vi "New Prop B.vi"(11 "GIC Input":T1={"     Use ?\nOff       On"=[FALSE, TRUE, FALSE, TRUE], "Mode:"=FALSE, "WP Data"="", "Hokuyo Port"="COM7", "Prop  Port"="COM6", "Compass Port"="", "GPS Port"="", "Num of WPs"=0, "WP Lats and Longs"={"WP Lats"=[], "WP Longs"=[]}, "Obst Lats and Longs"={"Obst Lats"=[], "Obst Longs"=[]}, "Parameters"=[], "GPS Data"=[], "Compass"=0.0, "LMS Vector"=[], "Vision Vector"=[], "Direction Cmd"=0.0, "Speed Cmd"=0.0, "WP Vector"=[], "WP Number"=0, "Extra"=0, "SW Map"=[], "Path Cluster"={"Path x node"=[], "Path y node"=[]}} {"Obst Lats and Longs"."Obst Longs" format="%#_8g"; "Obst Lats and Longs"."Obst Lats" format="%#_8g"}) -> ()   [LabVIEW 2014]
uses:
  <vilib>/Instr/_visa.llb/VISA Configure Serial Port (Instr).vi
panel:
  out "Prop VISA Resource Name":refnum<visa-resource-name>
  # "New Prop B"
  # "Input:"
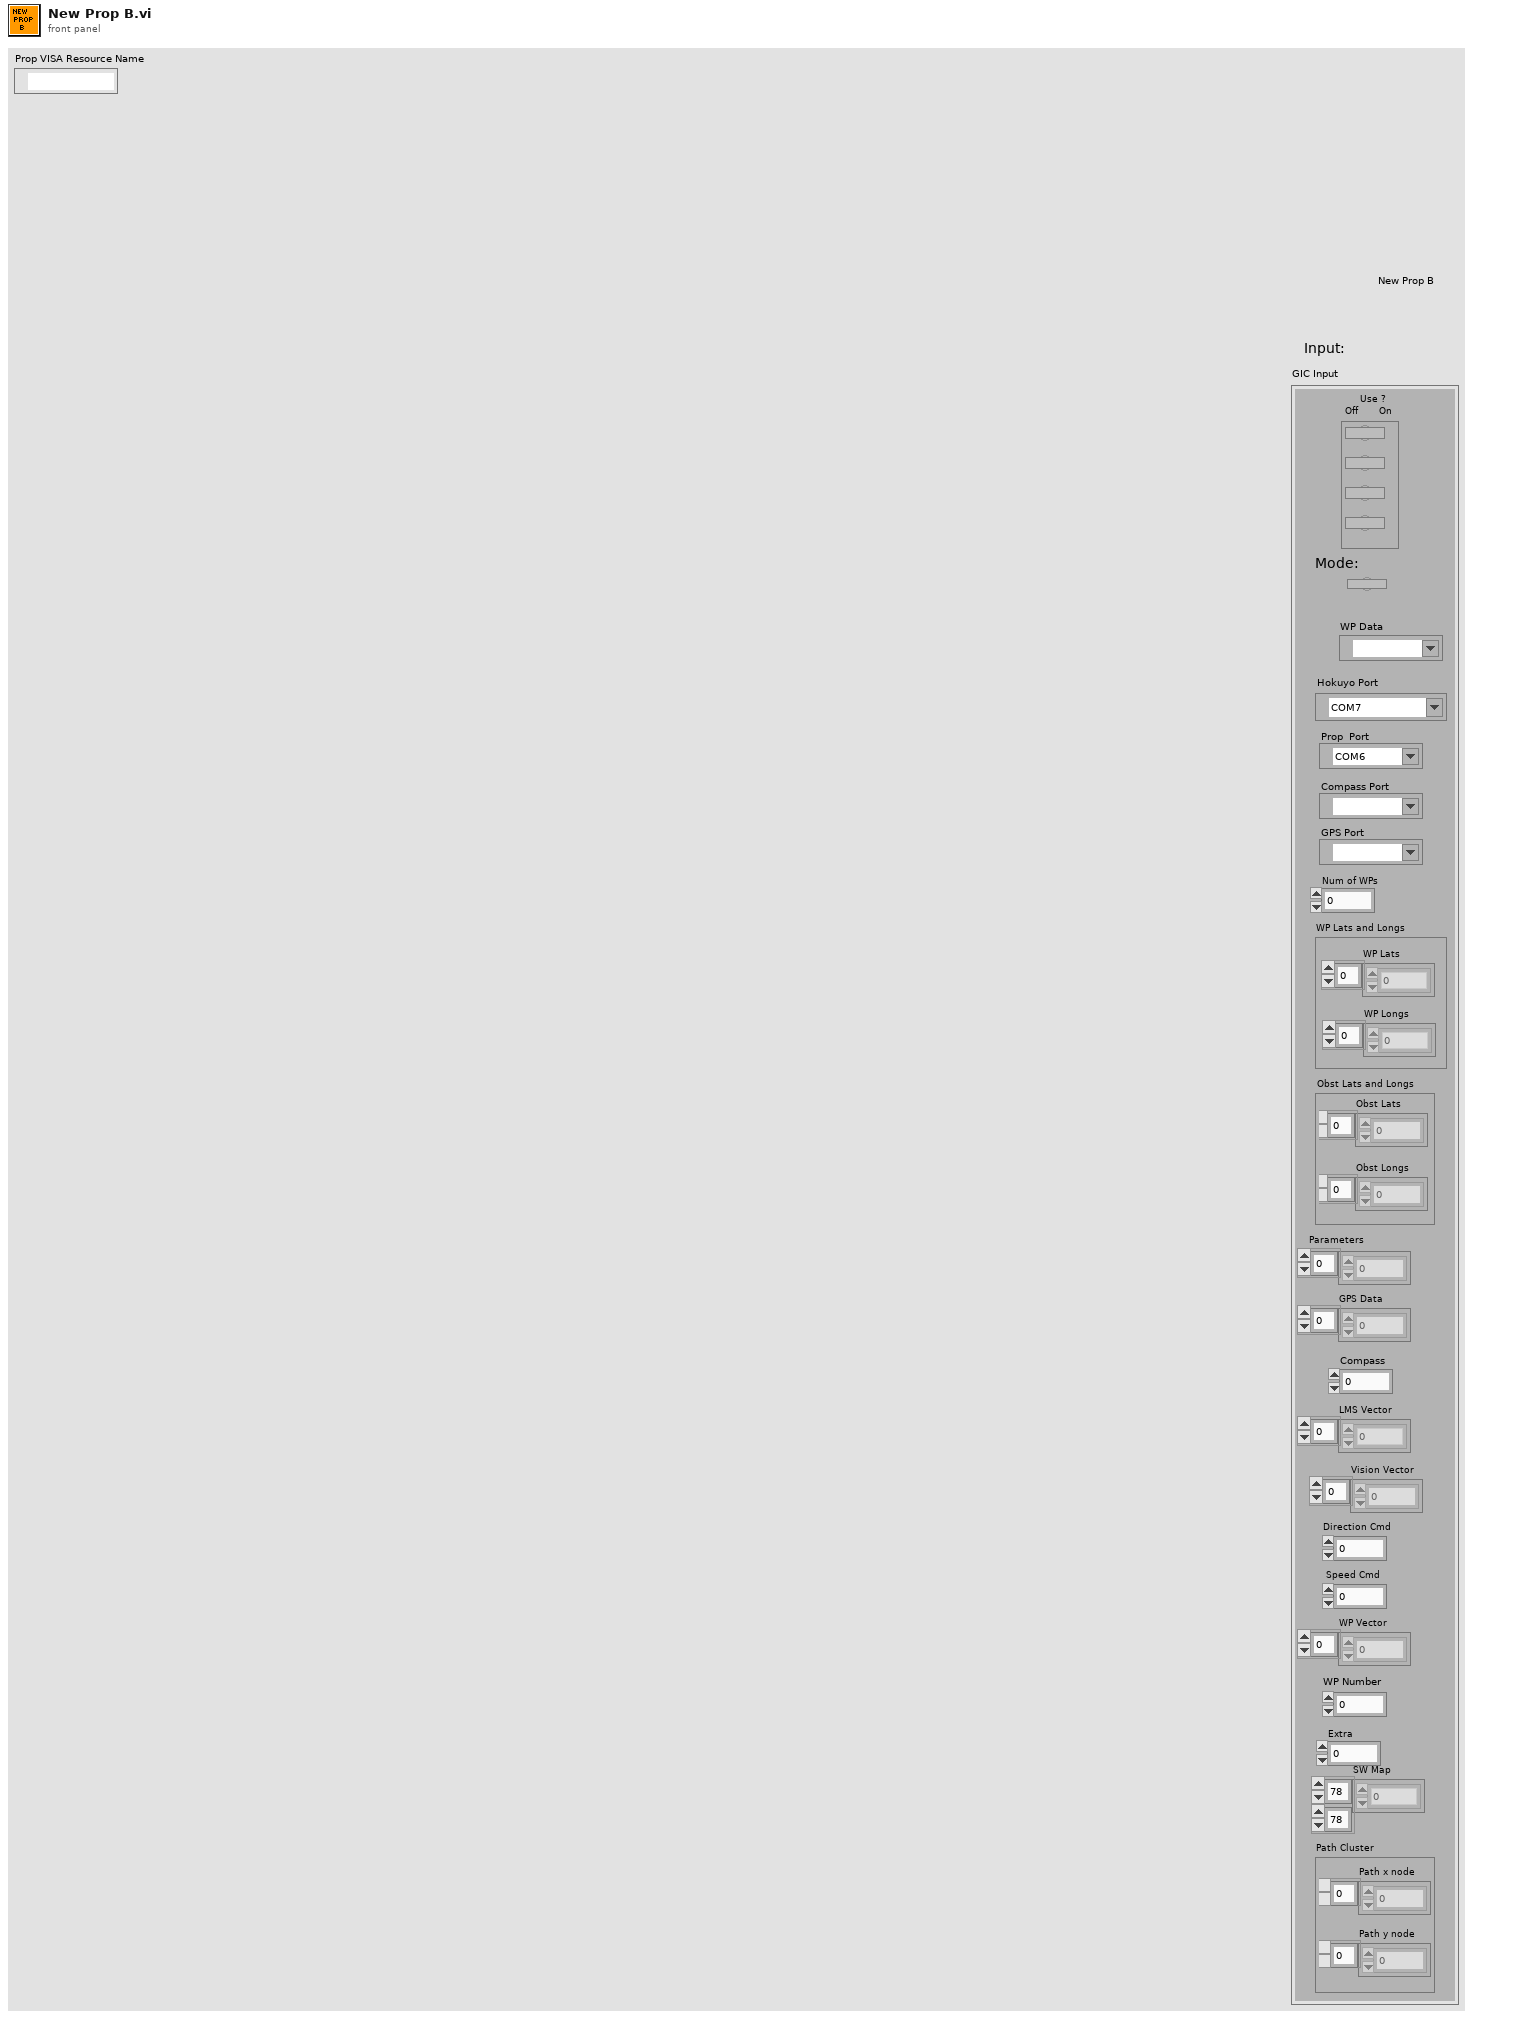
[diagram p1: front panel]
types:
  T1 = cluster{"     Use ?\nOff       On":bool[], "Mode:":bool, "WP Data":refnum<visa-resource-name>, "Hokuyo Port":refnum<visa-resource-name>, "Prop  Port":refnum<visa-resource-name>, "Compass Port":refnum<visa-resource-name>, "GPS Port":refnum<visa-resource-name>, "Num of WPs":i16, "WP Lats and Longs":cluster{"WP Lats":dbl[], "WP Longs":dbl[]}, "Obst Lats and Longs":cluster{"Obst Lats":dbl[], "Obst Longs":dbl[]}, "Parameters":dbl[], "GPS Data":dbl[], "Compass":dbl, "LMS Vector":dbl[], "Vision Vector":dbl[], "Direction Cmd":dbl, "Speed Cmd":dbl, "WP Vector":dbl[], "WP Number":i32, "Extra":i16, "SW Map":i32[][], "Path Cluster":cluster{"Path x node":dbl[], "Path y node":dbl[]}}
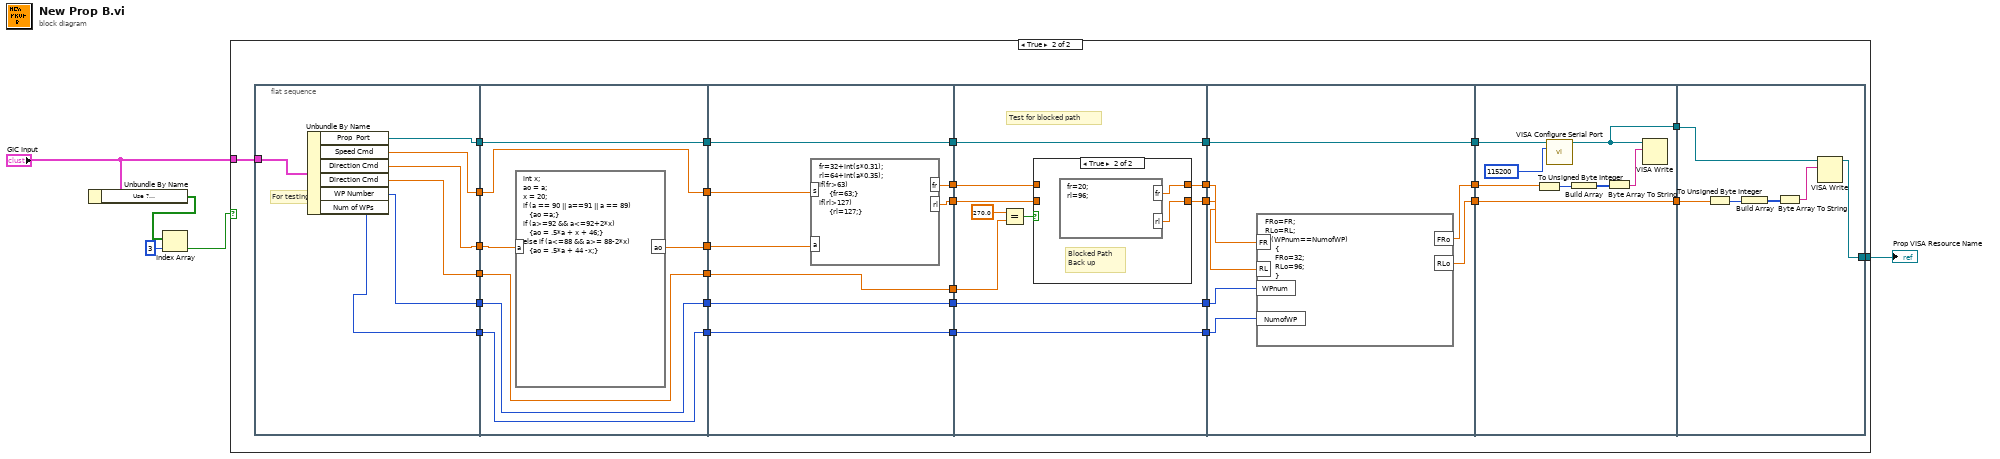
[diagram p0: block diagram]
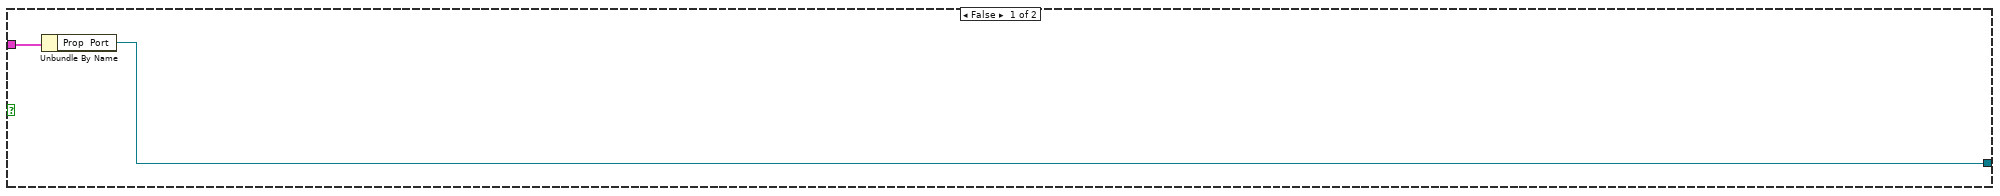
[diagram p2: hidden frame]
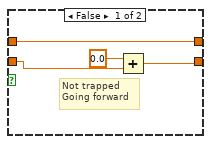
[diagram p3: hidden frame]
diagram:
  n1 = Unbundle By Name("GIC Input") -> ("Use ?\nOff       On"=w5:bool[])
  n2 = Index Array(array=w5, index=3) -> (element=w3:bool)
  n3 = case shown="True" w3 {
    tunnel: "GIC Input" -> [w7 w31]
    tunnel: [w6 w20] -> w2
    frame False {
      n4 = Unbundle By Name(w7) -> ("Prop  Port"=w6:refnum<visa-resource-name>)
    }
    frame True {
      n5 = flat-sequence {
        tunnel: [w44] -> w13
        tunnel: [w43] -> w15
        tunnel: [w42] -> w17
        tunnel: [w41] -> w19
        tunnel: w31 -> [w40]
        tunnel: [w39] -> w11
        tunnel: [w38] -> w9
        tunnel: w19 -> [w47]
        tunnel: [w47] -> w18
        tunnel: w17 -> [w46]
        tunnel: [w45] -> w16
        tunnel: w15 -> [w50]
        tunnel: [w50] -> w14
        tunnel: w13 -> [w51]
        tunnel: [w51] -> w12
        tunnel: w11 -> [w48]
        tunnel: [w48] -> w10
        tunnel: w9 -> [w49]
        tunnel: [w49] -> w8
        tunnel: [w59] -> w37
        tunnel: [w56] -> w36
        tunnel: [w55] -> w35
        tunnel: [w54] -> w34
        tunnel: w18 -> [w54]
        tunnel: w16 -> [w57]
        tunnel: w14 -> [w58]
        tunnel: w12 -> [w59]
        tunnel: [w53] -> w23
        tunnel: w10 -> [w53]
        tunnel: [w52] -> w21
        tunnel: w8 -> [w52]
        tunnel: w37 -> [w69]
        tunnel: [w69] -> w30
        tunnel: w36 -> [w65]
        tunnel: [w64] -> w28
        tunnel: w35 -> [w63]
        tunnel: [w62] -> w26
        tunnel: w34 -> [w66]
        tunnel: [w61] -> w24
        tunnel: w23 -> [w61]
        tunnel: [w60] -> w22
        tunnel: w21 -> [w60]
        tunnel: w30 -> [w82]
        tunnel: [w82] -> w29
        tunnel: w28 -> [w81]
        tunnel: [w79] -> w27
        tunnel: w26 -> [w80]
        tunnel: [w78] -> w25
        tunnel: w24 -> [w77]
        tunnel: w22 -> [w76]
        tunnel: [w86] -> w33
        tunnel: w29 -> [w85]
        tunnel: w27 -> [w84]
        tunnel: [w83] -> w32
        tunnel: w25 -> [w83]
        tunnel: w33 -> [w93]
        tunnel: w32 -> [w92]
        tunnel: [w91] -> w20
        frame #0 {
          # "For testing:"
          n6 = Unbundle By Name(w40) -> ("Prop  Port"=w44:refnum<visa-resource-name>, "Speed Cmd"=w43:dbl, "Direction Cmd"=w42:dbl, "Direction Cmd"=w41:dbl, "WP Number"=w39:i32, "Num of WPs"=w38:i16)
        }
        frame #1 {
          n7 = formula code="int x;\nao = a;\nx = 20;\nif (a == 90 || a==91 || a == 89)\n   {ao =a;}\nif (a>=92 && a<=92+2*x)\n   {ao = .5*a + x + 46;}\nelse if (a<=88 && a>= 88-2*x)\n   {ao = .5*a + 44 -x;}"("a"=w46) -> ("ao"=w45:dbl)
        }
        frame #2 {
          n8 = formula code="fr=32+int(s*0.31);\nrl=64+int(a*0.35);\nif(fr>63)\n     {fr=63;}\nif(rl>127)\n     {rl=127;}"("s"=w58, "a"=w57) -> ("fr"=w56:dbl, "rl"=w55:dbl)
        }
        frame #3 {
          # "Test for blocked path"
          n9 = Equal?(x=270.0, y=w66) -> (x = y?=w68:bool)
          n10 = case shown="True" w68 {
            tunnel: w65 -> [w73 _]
            tunnel: [w73 w75] -> w64
            tunnel: w63 -> [w71 _]
            tunnel: [w72 w74] -> w62
            frame False {
              # "Not trapped\nGoing forward"
              n11 = Add(x=0.0, y=w71) -> (x+y=w72:dbl)
            }
            frame True {
              # "Blocked Path\nBack up"
              n12 = formula code="fr=20;\nrl=96;"() -> ("fr"=w75:dbl, "rl"=w74:dbl)
            }
          }
        }
        frame #4 {
          n13 = formula code="FRo=FR;\nRLo=RL;\nif (WPnum==NumofWP)\n     {\n     FRo=32;\n     RLo=96;\n     }"("FR"=w81, "RL"=w80, "WPnum"=w77, "NumofWP"=w76) -> ("FRo"=w79:dbl, "RLo"=w78:dbl)
        }
        frame #5 {
          n14 = To Unsigned Byte Integer(number=w84) -> (unsigned 8bit integer=w88:u8)
          n15 = call-poly "VISA Configure Serial Port"("VISA resource name"=w85, "baud rate (9600)"=115200) -> ("VISA resource name out"=w86:refnum<visa-resource-name>)  [unwired: 12 in, 1 out]
          n16 = Build Array(w88) -> (w87:u8[])
          n17 = Byte Array To String(unsigned byte array=w87) -> (string=w89:string)
          n18 = VISA Write(VISA resource name=w86, write buffer=w89) -> ()  [unwired: 1 in, 3 out]
        }
        frame #6 {
          n19 = To Unsigned Byte Integer(number=w92) -> (unsigned 8bit integer=w95:u8)
          n20 = Build Array(w95) -> (w96:u8[])
          n21 = Byte Array To String(unsigned byte array=w96) -> (string=w94:string)
          n22 = VISA Write(VISA resource name=w93, write buffer=w94) -> (VISA resource name out=w91:refnum<visa-resource-name>)  [unwired: 1 in, 2 out]
        }
      }
    }
  }
  "Prop VISA Resource Name" <- w2
